vi "RT-Config.vi"(10 "Target Name":string) -> (2 "IP Address":string, 3 "Target (Detected)":string)   [LabVIEW 2018]
panel:
  in  "OK":bool
  # "RT Target  Configuration"
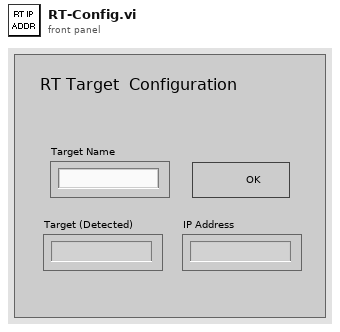
[diagram p1: front panel]
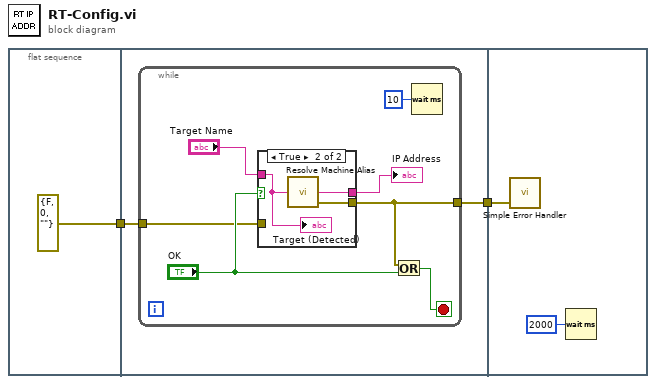
[diagram p0: block diagram]
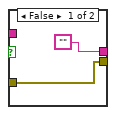
[diagram p2: hidden frame]
diagram:
  n1 = flat-sequence {
    tunnel: [errorcluster {"status"=FALSE, "code"=0, "source"=""} ("error constant")] -> w2
    tunnel: w2 -> [w5]
    tunnel: [w4] -> w1
    tunnel: w1 -> [w18]
    frame #0 {
    }
    frame #1 {
      n2 = while {
        tunnel: w5 -> [w8]
        tunnel: [w7] -> w4
        stop <- w11 stop-if-true
        n3 = case shown="True" "OK" {
          tunnel: [w13 w17] -> w7
          tunnel: ["" w16] -> w10
          tunnel: "Target Name" -> [_ w15]
          tunnel: w8 -> [w13 _]
          frame False {
          }
          frame True {
            n4 = call <vilib>:"Resolve Machine Alias.vi"("Machine Alias"=w15) -> ("error out"=w17:errorcluster, "Network Identity"=w16:string)  [unwired: 2 in, 1 out]
            "Target (Detected)" <- w15
          }
        }
        "IP Address" <- w10
        n5 = Or(x=w7, y="OK") -> (x .or. y?=w11:bool)
        n6 = Wait (ms)(milliseconds to wait=u32 10) -> ()  [unwired: 1 out]
      }
    }
    frame #2 {
      n7 = call <vilib>:"Simple Error Handler.vi"("error in (no error)"=w18) -> ()  [unwired: 4 in, 5 out]
      n8 = Wait (ms)(milliseconds to wait=u32 2000) -> ()  [unwired: 1 out]
    }
  }
